vi "choice_band.vi"(7 "Master Volume":dbl, 8 "Mid tone":dbl, 9 "Treble":dbl, 10 "Bass":dbl, 11 "input waveform":waveform(dbl)) -> (3 "output waveform":waveform(dbl))   [LabVIEW 2024]
uses:
  <vilib>/Analysis/3filter.llb/Filter Passband Type.ctl
  <vilib>/Analysis/3filter.llb/Chebyshev Filter (DBL).vi
  <vilib>/Analysis/NI_AALBase.lvlib
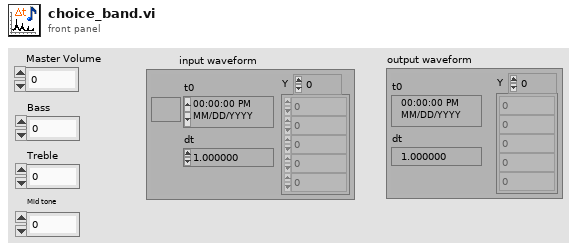
[diagram p1: front panel]
types:
  T1 = typedef "NI_AALBase.lvlib/Filter Passband Type.ctl" = enum32{"Lowpass", "Highpass", "Bandpass", "Bandstop"}
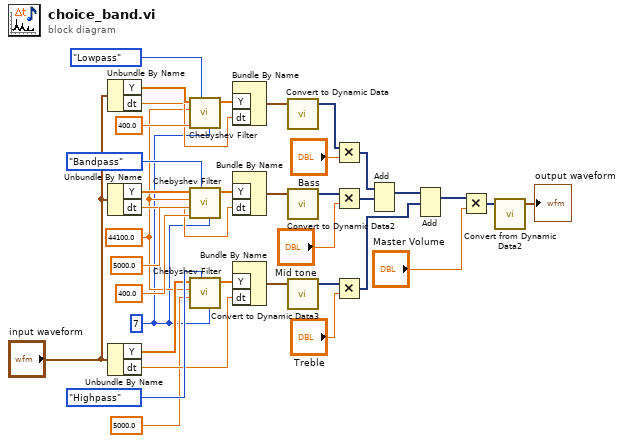
[diagram p0: block diagram]
diagram:
  w1 = 7 ("order")
  w3 = 44100.0 ("sampling freq: fs")
  n1 = Unbundle By Name("input waveform") -> ("Y"=w23:dbl[], "dt"=w21:dbl)
  n2 = Unbundle By Name("input waveform") -> ("Y"=w18:dbl[], "dt"=w14:dbl)
  n3 = Unbundle By Name("input waveform") -> ("Y"=w8:dbl[], "dt"=w5:dbl)
  n4 = call-poly <vilib>:"Chebyshev Filter.vi"("order"=w1, "filter type"=Filter_Passband_Type."Lowpass", "low cutoff freq: fl"=400.0, "sampling freq: fs"=w3, "X"=w23) -> ("Filtered X"=w22:dbl[])  [unwired: 5 in, 1 out]
  n5 = call-poly <vilib>:"Chebyshev Filter.vi"("order"=w1, "filter type"=Filter_Passband_Type."Bandpass", "low cutoff freq: fl"=400.0, "high cutoff freq: fh"=5000.0, "sampling freq: fs"=w3, "X"=w18) -> ("Filtered X"=w13:dbl[])  [unwired: 4 in, 1 out]
  n6 = call-poly <vilib>:"Chebyshev Filter.vi"("order"=w1, "filter type"=Filter_Passband_Type."Highpass", "high cutoff freq: fh"=5000.0, "sampling freq: fs"=w3, "X"=w8) -> ("Filtered X"=w4:dbl[])  [unwired: 5 in, 1 out]
  n7 = Bundle By Name("Y"=w22, "dt"=w21) -> (w20:waveform(dbl))  [unwired: 1 in]
  n8 = Bundle By Name("Y"=w13, "dt"=w14) -> (w12:waveform(dbl))  [unwired: 1 in]
  n9 = Bundle By Name("Y"=w4, "dt"=w5) -> (w7:waveform(dbl))  [unwired: 1 in]
  n10 = call "Convert to Dynamic Data"("Waveform"=w20) -> ("Dynamic Data Type"=w19:dynamicdata)  [unwired: 3 in]
  n11 = call "Convert to Dynamic Data2"("Waveform"=w12) -> ("Dynamic Data Type"=w11:dynamicdata)  [unwired: 3 in]
  n12 = call "Convert to Dynamic Data3"("Waveform"=w7) -> ("Dynamic Data Type"=w6:dynamicdata)  [unwired: 3 in]
  n13 = Multiply(x=w19, y="Bass") -> (x*y=w31:dynamicdata)
  n14 = Multiply(x=w11, y="Mid tone") -> (x*y=w34:dynamicdata)
  n15 = Multiply(x=w6, y="Treble") -> (x*y=w30:dynamicdata)
  n16 = Add(1:w34, 2:w31) -> (0:w32:dynamicdata)  [unwired: 1 in, 1 out]
  n17 = Add(1:w30, 2:w32) -> (0:w27:dynamicdata)  [unwired: 1 in, 1 out]
  n18 = Multiply(x=w27, y="Master Volume") -> (x*y=w26:dynamicdata)
  n19 = call "Convert from Dynamic Data2"("Dynamic Data Type"=w26) -> ("Waveform"=→"output waveform":waveform(dbl))  [unwired: 3 in]
